vi "MeasurementType.Edit.vi"(7 "Max Shots":T1(ring)=enum."1", 8 "error in (no error)":errorcluster, 9 "Stages":string[](array[string])=["Boost", "Battery", "Off"], 11 "Item Ref in":T2 format="%.0x") -> (0 "error out":errorcluster)   [LabVIEW 2015, in "Fuel Injector Analysis Addon System Explorer.lvlib"]
uses:
  Fuel Injector Analysis Addon System Explorer.lvlib
  <vilib>/NI Veristand/Custom Device API/Custom Device Item Ref.ctl
  Shared/Constants.vi
  <vilib>/NI Veristand/Custom Device API/Get Item Property (Path).vi
  Shared/Fuel Injector Analysis Addon Shared.lvlib
  <vilib>/NI Veristand/Custom Device API/Custom Device API.lvlib
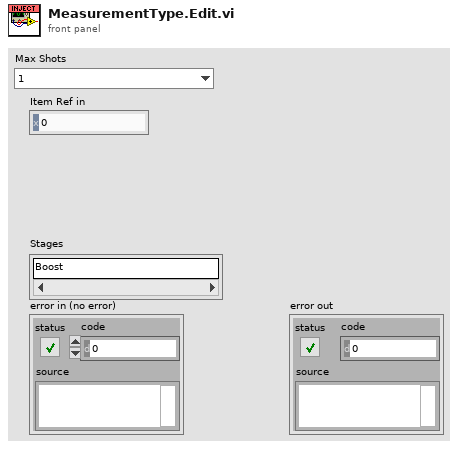
[diagram p1: front panel]
types:
  T1 = enum16{"0", "1", "2", "3", "4", "5", "6", "7", "8"}
  T2 = typedef "Custom Device API.lvlib/Custom Device Item Ref.ctl" = u64
  T3 = typedef "Fifo_DMA_Config.ctl" = cluster{"Name":string, "Depth":u32, "Write? (Deprecated:Use Implementation)":bool, "Physical Channel":u32, "Base Address":u32, "Data Width":u32, "Data Type":T4, "FXP Properties":variant, "Write Window Address":u32, "Implementation":T5, "Control Set":u32}
  T4 = typedef "niFpgaDataTypeControl.ctl" = enum32{"Boolean", "I8", "I16", "I32", "I64", "U8", "U16", "U32", "U64", "FXP", "CustomControl", "SGL"}
  T5 = typedef "niFpgaDmaChannelImplementation.ctl" = enum16{"niFpgaTargetToHost", "niFpgaHostToTarget", "niFpgaPeerToPeerWriter", "niFpgaPeerToPeerReader", "niCoreTargetToHost", "niCoreHostToTarget"}
  T6 = typedef "niFpgaBitfileStructure_VI.ctl" = cluster{"Name":string, "RegisterMap":T7[], "Icon":T12}
  T7 = typedef "nirviControlStructure.ctl" = cluster{"Name":string, "Hidden":bool, "Indicator":bool, "Flattened Type":string, "Grouping":cluster{"Grouped":bool, "Member Names":string[], "Member IDs":u32[]}, "Address":u32, "Size":u32, "Class":u32, "Internal":bool, "Typedef":T8, "ID":u32, "Bidirectional":bool, "Synchronous":bool, "Mechanical Action":T9, "Sub Controls":T10[], "Access May Timeout":bool, "Register Node":bool}
  T8 = typedef "nirviTypdefDescription.ctl" = cluster{"Typedef":bool, "Path":path}
  T9 = typedef "nirviMechanicalAction.ctl" = enum8{"Switch When Pressed", "Switch When Released", "Switch Until Released", "Latch When Pressed", "Latch When Released", "Latch Until Released"}
  T10 = typedef "nirviSubControlStructure.ctl" = cluster{"Name":string, "flattened Type":string, "Cluster Information":T11, "Typedef":T8}
  T11 = typedef "nirviClusterElementControl.ctl" = cluster{"Name Hierarchy":string[], "Item Order":u32[]}
  T12 = typedef "imagedata.ctl" = cluster{"image type":i32, "image depth":i32, "image":u8[], "mask":u8[], "colors":u32[], "Rectangle":cluster{"left":i16, "top":i16, "right":i16, "bottom":i16}}
  T13 = typedef "Fuel Injector Analysis Addon Shared.lvlib/Register.Info.ctl" = cluster{"Name":string, "Data Type":T14, "Default Value":variant}
  T14 = typedef "Fuel Injector Analysis Addon Shared.lvlib/FPGA Data Types.ctl" = enum8{"<Null>", "Injector.Core.Setting", "Injector.Global.Setting", "Injector.Mux.Setting", "Injector.Timing"}
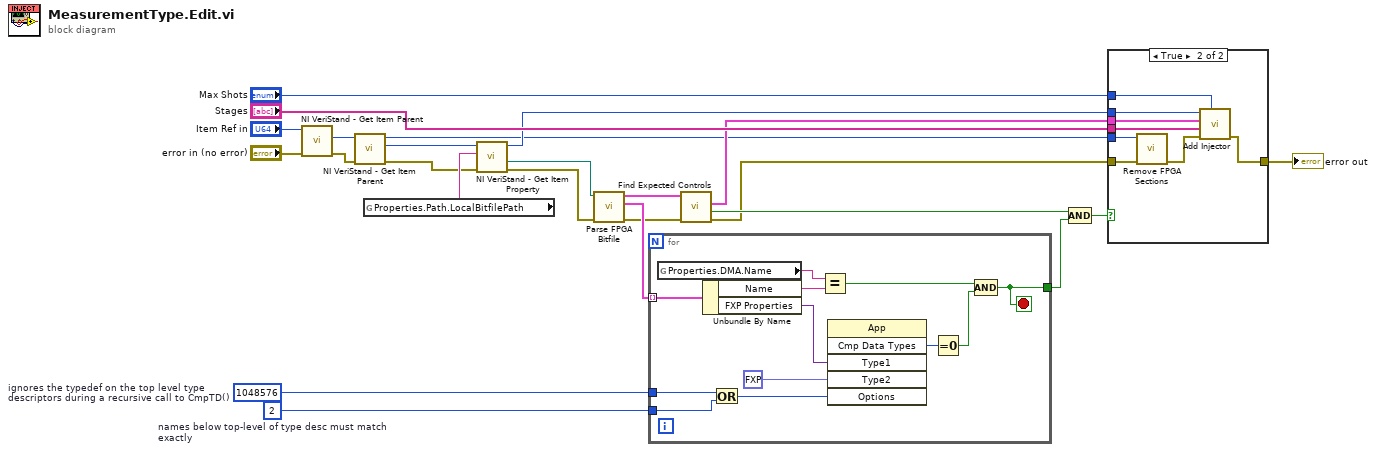
[diagram p0: block diagram]
diagram:
  w20 = 2  # names below top-level of type desc must match exactly
  w21 = 1048576  # ignores the typedef on the top level type descriptors during a recursive call to CmpTD()
  n1 = call <vilib>:"NI VeriStand - Get Item Parent.vi"("error in (no error)"="error in (no error)", "Item Ref in"="Item Ref in") -> ("error out"=w6:errorcluster, "Parent Ref"=w8:T2)  [unwired: 6 in, 2 out]
  n2 = call <vilib>:"NI VeriStand - Get Item Parent.vi"("error in (no error)"=w6, "Item Ref in"=w8) -> ("error out"=w5:errorcluster, "Parent Ref"=w7:T2, "Item Ref out"=w1:T2)  [unwired: 6 in, 1 out]
  n3 = global read "Constants.vi" "Properties.Path.LocalBitfilePath"() -> (w9:string)
  n4 = call-poly <vilib>:"NI VeriStand - Get Item Property.vi"("error in (no error)"=w5, "Property Name"=w9, "Item Ref in"=w7) -> ("error out"=w3:errorcluster, "Value"=w2:path, "Item Ref out"=w4:T2)  [unwired: 5 in, 1 out]
  n5 = call "Parse FPGA Bitfile.vi"("error in (no error)"=w3, "Path"=w2) -> ("error out"=w13:errorcluster, "DMA configuration array"=w15:T3[], "vi info"=w14:T6)  [unwired: 7 in]
  n6 = for {
    tunnel: w15 -> [w36] mode=indexing
    tunnel: [w32] -> w17
    tunnel: w21 -> [w27]
    tunnel: w20 -> [w26]
    stop <- w32 stop-if-true
    n7 = global read "Constants.vi" "Properties.DMA.Name"() -> (w34:string)
    n8 = Unbundle By Name(w36) -> ("Name"=w35:string, "FXP Properties"=w25:variant)
    n9 = Or(x=w27, y=w26) -> (x .or. y?=w31:i32)
    n10 = Equal?(x=w34, y=w35) -> (x = y?=w33:bool)
    n11 = invoke class="App" method="Cmp Data Types"("Type1"=w25, "Type2"=fxp<+/-,32,8> 0.0, "Options"=w31) -> ("Compare Data Types"=w29:i32)  [unwired: 3 in, 5 out]
    n12 = Equal To 0?(x=w29) -> (x = 0?=w28:bool)
    n13 = Compound Arithmetic op=AND(w33, w28) -> (w32:bool)
  }
  n14 = call "Find Expected Controls.vi"("error in"=w13, "vi info"=w14) -> ("error out"=w12:errorcluster, "Use?"=w16:bool, "Controls"=w10:T13[])  [unwired: 6 in, 1 out]
  n15 = Compound Arithmetic op=AND(w16, w17) -> (w11:bool)
  n16 = case shown="True" w11 {
    tunnel: w1 -> [_ w39]
    tunnel: w12 -> [w37 w40]
    tunnel: [w37 w44] -> w24
    tunnel: w10 -> [_ w43]
    tunnel: "Stages" -> [_ w42]
    tunnel: "Max Shots" -> [_ w41]
    tunnel: w4 -> [_ w38]
    frame False {
    }
    frame True {
      n17 = call "Remove FPGA Sections.vi"("error in (no error)"=w40, "Item Ref in"=w39) -> ("error out"=w45:errorcluster)  [unwired: 8 in, 1 out]
      n18 = call "Add Injector.vi"("Max Shots"=w41, "error in (no error)"=w45, "Stages"=w42, "Controls"=w43, "Item Ref"=w38) -> ("error out"=w44:errorcluster)  [unwired: 5 in, 1 out]
    }
  }
  "error out" <- w24
